vi "ElevatorSim_exampleX.vi"() -> ()   [LabVIEW 2019]
uses:
  <vilib>/Rock Robotics/WPI/ThirdParty/JAS_Junk/TrajLib/DCMOTOR.CTL
  <vilib>/Rock Robotics/WPI/ThirdParty/JAS_Junk/TrajLib/LINEAR_SYSTEM.ctl
  <vilib>/Analysis/Matrix/Datatypes/RealMatrix.ctl
  <vilib>/Rock Robotics/WPI/ThirdParty/JAS_Junk/TrajLib/LINEAR_QUADRATIC_REGULATOR.ctl
  <vilib>/Rock Robotics/WPI/ThirdParty/JAS_Junk/TrajLib/KALMAN_FILTER.ctl
  <vilib>/Rock Robotics/WPI/ThirdParty/JAS_Junk/TrajLib/LINEAR_SYSTEM_LOOP.ctl
  <vilib>/Rock Robotics/WPI/ThirdParty/JAS_Junk/TrajLib/LINEAR_PLANT_INV_FF.ctl
  <vilib>/Rock Robotics/WPI/ThirdParty/JAS_Junk/TrajLib/ELEVATOR_SIM.ctl
  <vilib>/Rock Robotics/WPI/ThirdParty/JAS_Junk/TrajLib/LINEAR_SYSTEM_SIM.ctl
  <vilib>/numeric/Random Number (Range) DBL.vi
  <vilib>/Rock Robotics/WPI/ThirdParty/JAS_Junk/TrajLib/MatBuilder_Create.vi
  <vilib>/Rock Robotics/WPI/ThirdParty/JAS_Junk/TrajLib/DCMotor_New.vi
  <vilib>/Rock Robotics/WPI/ThirdParty/JAS_Junk/TrajLib/Units_RotationsPerMinuteToRadiansPerSecond.vi
  <vilib>/Rock Robotics/WPI/ThirdParty/JAS_Junk/TrajLib/MatBuilder_Fill.vi
  <vilib>/Rock Robotics/WPI/ThirdParty/JAS_Junk/TrajLib/MatrixHelper_Zero.vi
  <vilib>/Rock Robotics/WPI/ThirdParty/JAS_Junk/TrajLib/LinearSystem_New.vi
  <vilib>/Rock Robotics/WPI/ThirdParty/JAS_Junk/TrajLib/Trajectory_Library.lvlib
  <vilib>/Analysis/Matrix/NI_Matrix.lvlib
panel:
  in  "Tab Control":T1(tab)
  out "Elevator Motor":T2 {"Jr_KgM2" format="%13.5p"; "L_H" format="%13.5p"; "Kt_NMPerAmp" format="%13.5p"; "KvINV_RadPerSecPerVolt" format="%13.5p"; "R_Ohms" format="%13.5p"; "FreeSpeed_RadPerSec" format="%13.5p"; "FreeCurrent_Amps" format="%13.5p"; "StallCurrent_Amps" format="%13.5p"; "StallTorque_NM" format="%13.5p"; "nominalVoltage_Volts" format="%13.5p"}
  out "m_Elevator":T3
  out "KalmanFilter":T5
  out "Kalman Error":bool
  out "LinearQuadraticRegulator":T6
  out "LQR Error":bool
  out "Linear System Loop":T7
  out "LinSysLoop_Error":bool
  out "Elevator Simulaation":T9 {"GearBox"."Jr_KgM2" format="%13.5p"; "GearBox"."L_H" format="%13.5p"; "GearBox"."Kt_NMPerAmp" format="%13.5p"; "GearBox"."KvINV_RadPerSecPerVolt" format="%13.5p"; "GearBox"."R_Ohms" format="%13.5p"; "GearBox"."FreeSpeed_RadPerSec" format="%13.5p"; "GearBox"."FreeCurrent_Amps" format="%13.5p"; "GearBox"."StallCurrent_Amps" format="%13.5p"; "GearBox"."StallTorque_NM" format="%13.5p"; "GearBox"."nominalVoltage_Volts" format="%13.5p"}
  out "Shooting A":T4
  out "Shooting B":T4
  out "Battery Voltage":dbl format="%20.3f"
  in  "Extra weight":bool
  out "CO Chart":cluster{dbl, "Voltage":dbl}(graph)
  in  "GO UP":bool
  out "Encoer Speed\nRad/Sec":dbl(slide) scale=-1.0..6.0
  out "Height":dbl format="%20.3f"
  out "Cor Err":bool
  out "Kalman Filtered\nHeight":dbl format="%20.3f"
  out "PV Chart":T11(graph)
  out "Predict Err":bool
  out "Motor Volt Dmd (CO)":dbl format="%20.3f"
  out "At Top":bool
  out "At Bottom":bool
  out "Motor Amps":dbl format="%20.3f"
  # "<States,States>"
  # "<States,Inputs>"
  # "<Outputs,States>"
  # "<Outputs,Inputs>"
  # "Steady State Gain  \n<States,Outputs>"
  # "State Estimate <Statess,1>"
  # "<States,States>"
  # "<States,Inputs>"
  # "<Outputs,States>"
  # "<Outputs,Inputs>"
  # "Ref State <States,1>"
  # "Comp and capped \noutput <Inputs,1>"
  # "Controller gain\n<Inputs,States>"
  # "<States,1>"
  # "<FUTURE --- CLAMP TYPE -- For now\nuse Normalize>"
  # "Steady State Gain  \n<States,Outputs>"
  # "State Estimate <Statess,1>"
  # "<States,States>"
  # "<States,Inputs>"
  # "<Outputs,States>"
  # "<Outputs,Inputs>"
  # "<States,1>"
  # "<Inputs,1>"
  # "<States,Inputs>"
  # "<States,States>"
  # "Ref State <States,1>"
  # "Comp and capped \noutput <Inputs,1>"
  # "Controller gain\n<Inputs,States>"
  # "<States, 1>"
  # "<Outputs, 1>"
  # "<Inputs, 1>"
  # "<Outputs, 1>"
  # "<States,States>"
  # "<States,Inputs>"
  # "<Outputs,States>"
  # "<Outputs,Inputs>"
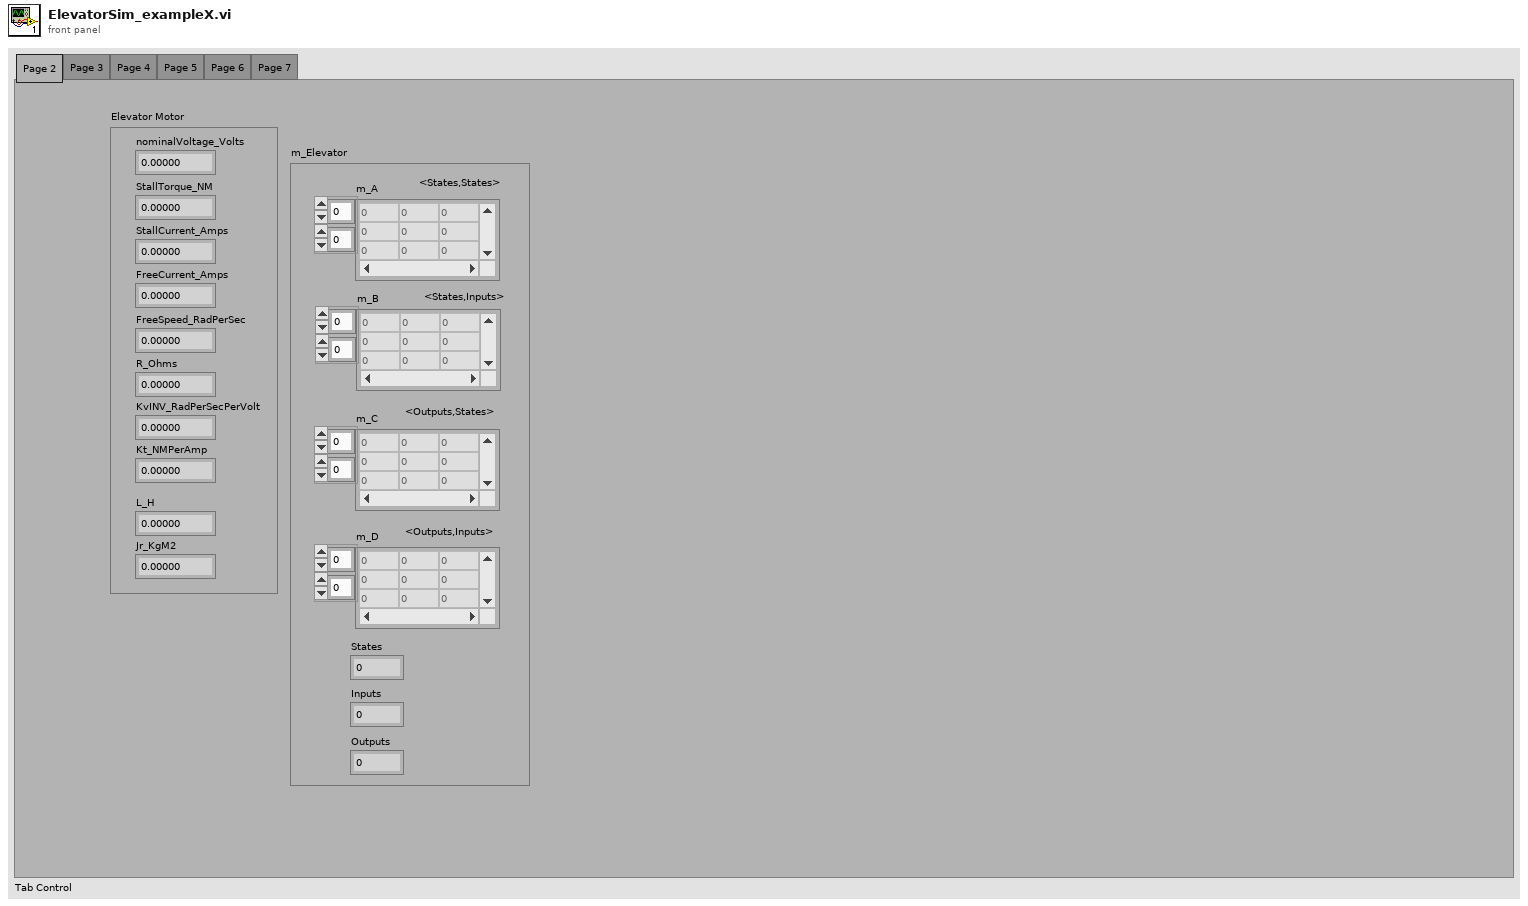
[diagram p1: front panel]
types:
  T1 = enum32{"Page 2", "Page 3", "Page 4", "Page 5", "Page 6", "Page 7"}
  T2 = typedef "Trajectory_Library.lvlib/DCMOTOR.CTL" = cluster{"nominalVoltage_Volts":dbl, "StallTorque_NM":dbl, "StallCurrent_Amps":dbl, "FreeCurrent_Amps":dbl, "FreeSpeed_RadPerSec":dbl, "R_Ohms":dbl, "KvINV_RadPerSecPerVolt":dbl, "Kt_NMPerAmp":dbl, "L_H":dbl, "Jr_KgM2":dbl}
  T3 = typedef "Trajectory_Library.lvlib/LINEAR_SYSTEM.ctl" = cluster{"m_A":T4, "m_B":T4, "m_C":T4, "m_D":T4, "States":i32, "Inputs":i32, "Outputs":i32}
  T4 = typedef "NI_Matrix.lvlib/RealMatrix.ctl" = dbl[][]
  T5 = typedef "Trajectory_Library.lvlib/KALMAN_FILTER.ctl" = cluster{"m_K":T4, "m_xHat":T4, "States":i32, "Outputs":i32, "m_Plant":T3}
  T6 = typedef "Trajectory_Library.lvlib/LINEAR_QUADRATIC_REGULATOR.ctl" = cluster{"m_r":T4, "m_U":T4, "m_K":T4, "States":i32, "Inputs":i32}
  T7 = typedef "Trajectory_Library.lvlib/LINEAR_SYSTEM_LOOP.ctl" = cluster{"Controller":T6, "FeedForward":T8, "Observer":T5, "Next_R":T4, "Clamp Max":T4}
  T8 = typedef "Trajectory_Library.lvlib/LINEAR_PLANT_INV_FF.ctl" = cluster{"m_R":T4, "m_Uff":T4, "m_B":T4, "m_A":T4, "States":i32, "Inputs":i32}
  T9 = typedef "Trajectory_Library.lvlib/ELEVATOR_SIM.ctl" = cluster{"LinearSystemSim":T10, "GearBox":T2, "Gearing":dbl, "DrumRadius_M":dbl, "MinHeight_M":dbl, "MaxHeight_M":dbl, "CarriageMass_Kg":dbl}
  T10 = typedef "Trajectory_Library.lvlib/LINEAR_SYSTEM_SIM.ctl" = cluster{"m_Plant":T3, "m_X":T4, "m_Y":T4, "m_U":T4, "MeasureStdDev":T4}
  T11 = cluster{"upper limit":dbl, "Real Matrix Element":dbl, "Real Matrix Element":dbl}
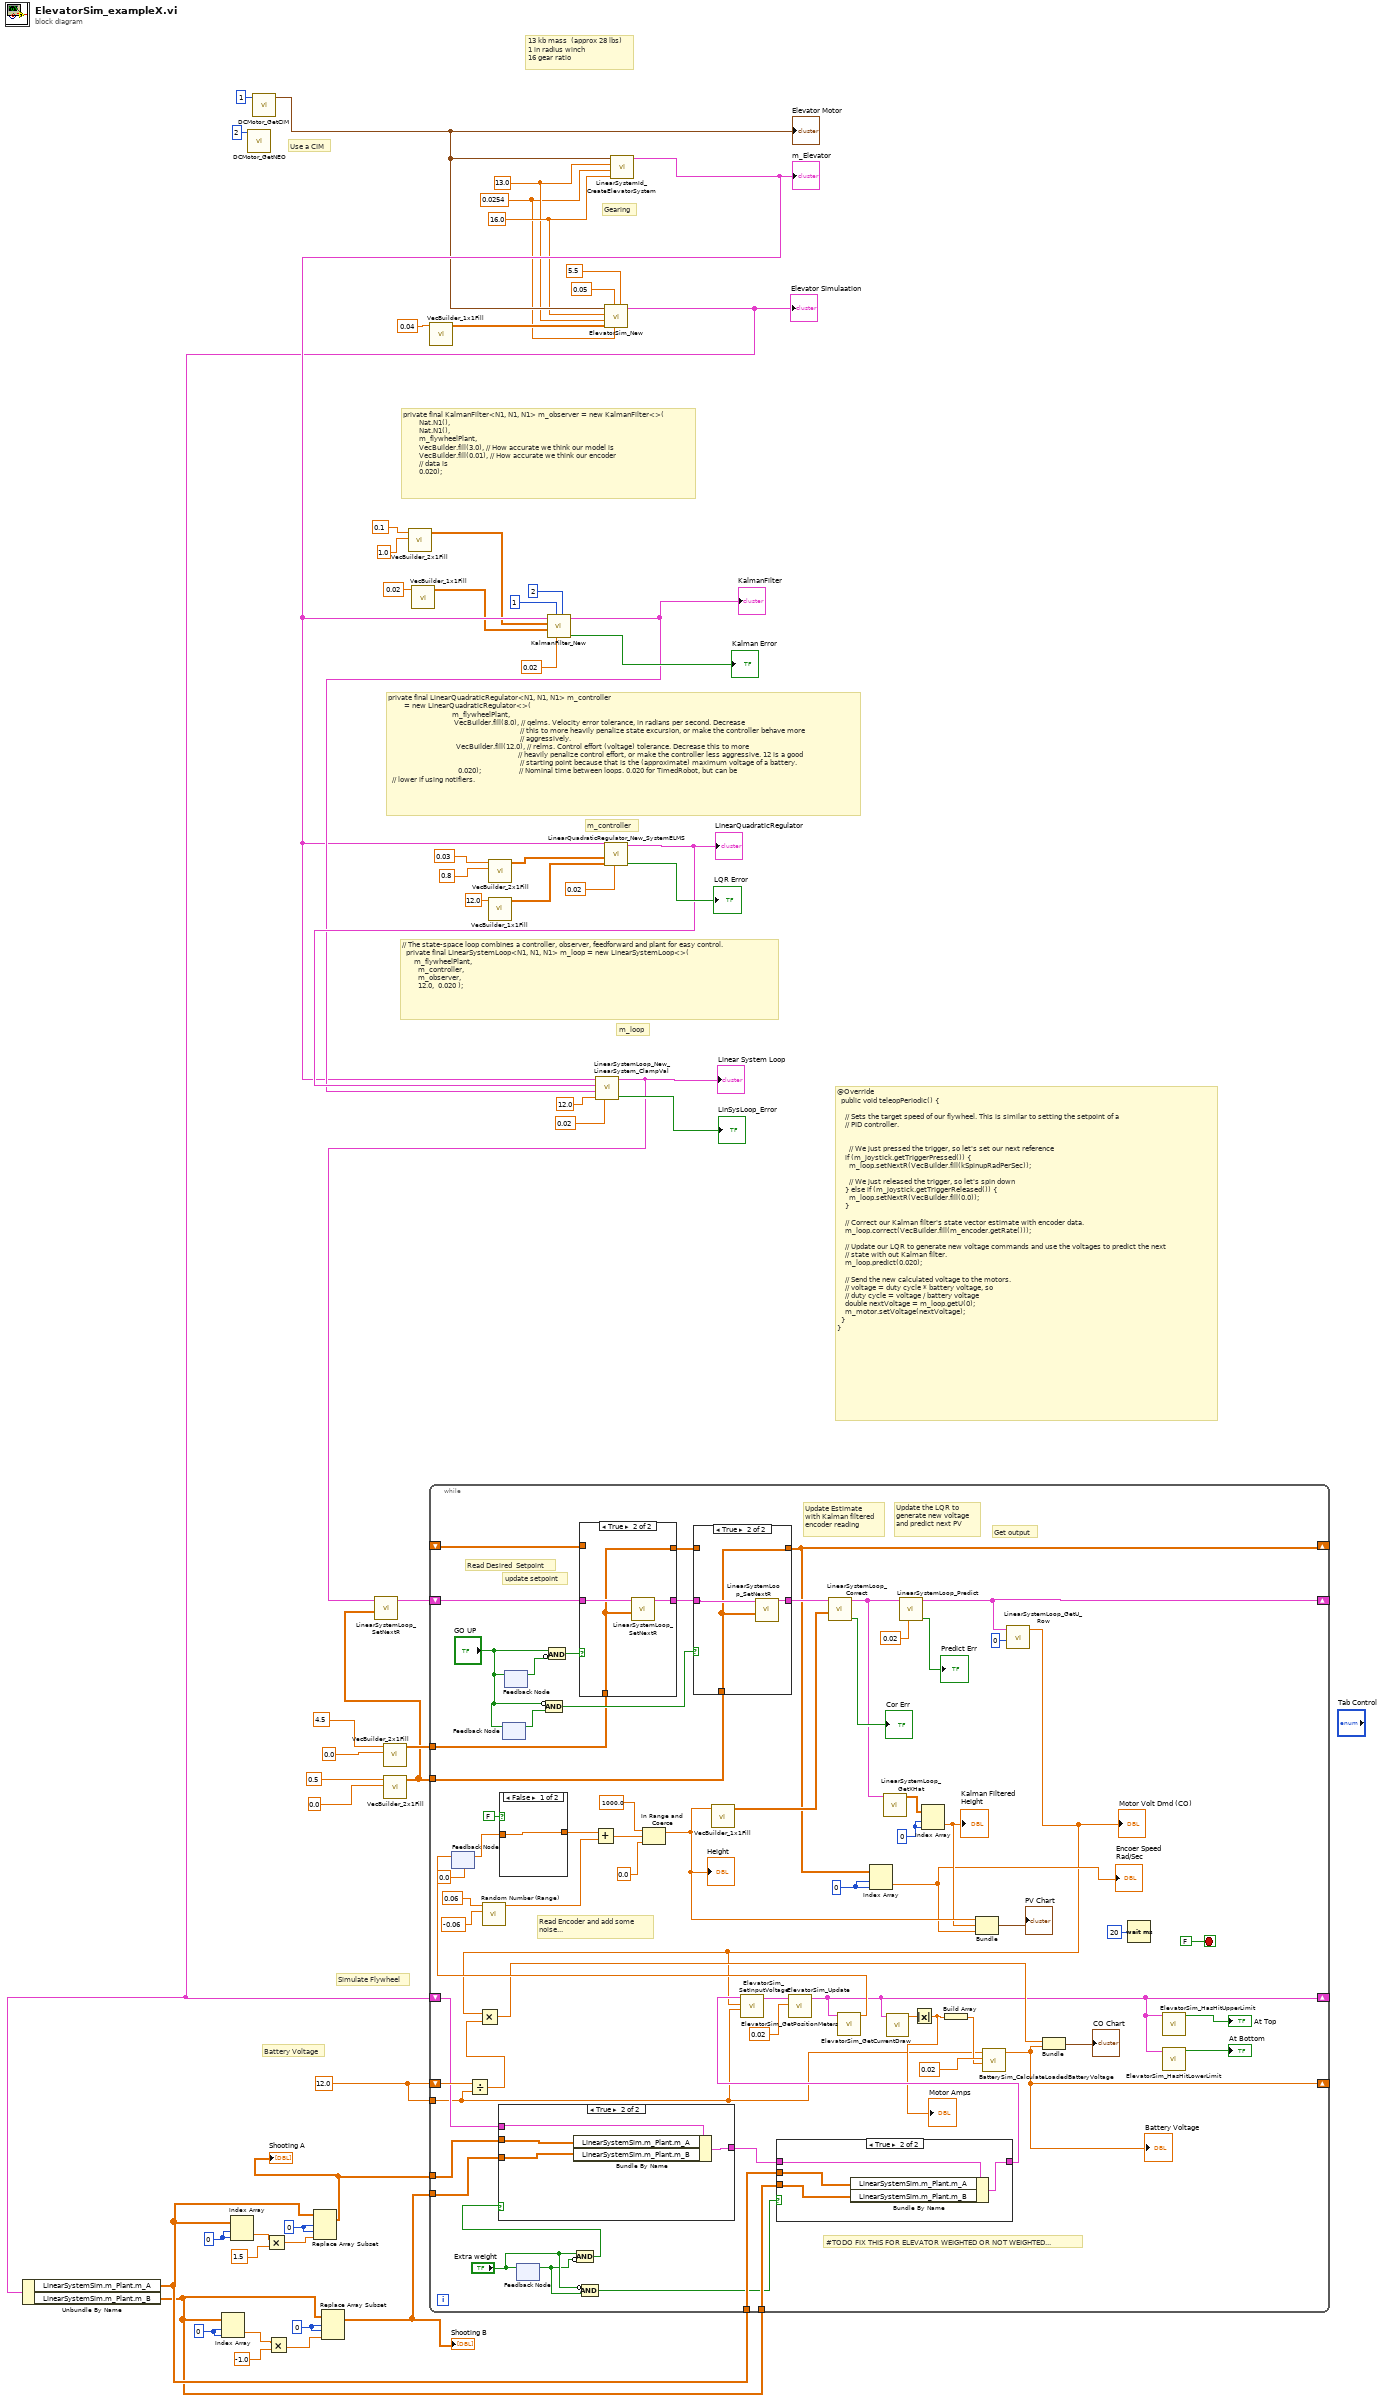
[diagram p0: block diagram]
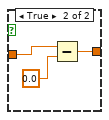
[diagram p4: hidden frame]
diagram:
  w13 = 0 ("index (row)")
  w14 = 0 ("index (row)")
  w15 = 0 ("index (row)")
  w16 = 0 ("index (row)")
  w36 = 16.0 ("G")
  w34 = 0.0254 ("radiusMeters")
  w35 = 13.0 ("massKg")
  w48 = 12.0
  # "Simulate Flywheel"
  # "m_loop"
  # "m_controller"
  # "13 kb mass  (approx 28 lbs)\n1 in radius winch\n16 gear ratio"
  # "Gearing"
  # "Use a CIM"
  # "Battery Voltage"
  # "@Override\n  public void teleopPeriodic() {\n\n    // Sets the target speed of our flywheel. This is similar to setting the setpoint of a\n    // PID controller.\n\n\n      // We just pressed the trigger, so let's set our next reference\n    if (m_joystick.getTriggerPressed()) {\n      m_loop.setNextR(VecBuilder.fill(kSpinupRadPerSec));\n\n      // We just released the trigger, so let's spin down\n    } else if (m_joystick.getTriggerReleased()) {\n      m_loop.setNextR(VecBuilder.fill(0.0));\n    }\n\n    // Correct our Kalman filter's state vector estimate with encoder data.\n    m_loop.correct(VecBuilder.fill(m_encoder.getRate()));\n\n    // Update our LQR to generate new voltage commands and use the voltages to predict the next\n    // state with out Kalman filter.\n    m_loop.predict(0.020);\n\n    // Send the new calculated voltage to the motors.\n    // voltage = duty cycle * battery voltage, so\n    // duty cycle = voltage / battery voltage\n    double nextVoltage = m_loop.getU(0);\n    m_motor.setVoltage(nextVoltage);\n  }\n}"
  # "// The state-space loop combines a controller, observer, feedforward and plant for easy control.\n  private final LinearSystemLoop<N1, N1, N1> m_loop = new LinearSystemLoop<>(\n      m_flywheelPlant,\n        m_controller,\n        m_observer,\n        12.0,  0.020 );"
  # "private final LinearQuadraticRegulator<N1, N1, N1> m_controller\n        = new LinearQuadraticRegulator<>(\n                                m_flywheelPlant,\n                                 VecBuilder.fill(8.0), // qelms. Velocity error tolerance, in radians per second. Decrease\n                                                                  // this to more heavily penalize state excursion, or make the controller behave more\n                                                                  // aggressively.\n                                  VecBuilder.fill(12.0), // relms. Control effort (voltage) tolerance. Decrease this to more\n                                                                 // heavily penalize control effort, or make the controller less aggressive. 12 is a good\n                                                                  // starting point because that is the (approximate) maximum voltage of a battery.\n                                   0.020);                   // Nominal time between loops. 0.020 for TimedRobot, but can be\n  // lower if using notifiers."
  # "private final KalmanFilter<N1, N1, N1> m_observer = new KalmanFilter<>(\n        Nat.N1(), \n        Nat.N1(),\n        m_flywheelPlant,\n        VecBuilder.fill(3.0), // How accurate we think our model is\n        VecBuilder.fill(0.01), // How accurate we think our encoder\n        // data is\n        0.020);"
  n1 = call <vilib>:"DCMotor_GetNEO.vi"("Num Motors"=2) -> ()  [unwired: 10 in, 1 out]
  n2 = call <vilib>:"DCMotor_GetCIM.vi"("Num Motors"=1) -> ("DCMOTOR"=w41:T2)  [unwired: 10 in]
  "Elevator Motor" <- w41
  n3 = call <vilib>:"VecBuilder_2x1Fill.vi"("R1"=0.0, "R0"=4.5 ("RotationsPerMinute")) -> ("output matrix"=w6:T4)  [unwired: 9 in]
  n4 = call <vilib>:"VecBuilder_2x1Fill.vi"("R1"=0.0, "R0"=0.5 ("R0_C0")) -> ("output matrix"=w1:T4)  [unwired: 9 in]
  n5 = call <vilib>:"VecBuilder_2x1Fill.vi"("R1"=1.0, "R0"=0.1 ("R0_C0")) -> ("output matrix"=w27:T4)  [unwired: 9 in]
  n6 = call <vilib>:"VecBuilder_1x1Fill.vi"("R0_C0"=0.02) -> ("output matrix"=w26:T4)  [unwired: 10 in]
  n7 = call <vilib>:"VecBuilder_1x1Fill.vi"("R0_C0"=0.04) -> ("output matrix"=w37:T4)  [unwired: 10 in]
  n8 = call <vilib>:"VecBuilder_1x1Fill.vi"("R0_C0"=12.0) -> ("output matrix"=w20:T4)  [unwired: 10 in]
  n9 = call <vilib>:"VecBuilder_2x1Fill.vi"("R1"=0.8 ("R0_C0"), "R0"=0.03 ("R0_C0")) -> ("output matrix"=w22:T4)  [unwired: 9 in]
  n10 = call <vilib>:"ElevatorSim_New.vi"("MaxHeight_Meters"=5.5, "DrumRadius_Meters"=w34, "MinHeight_Meters"=0.05, "MeasurementStdDev"=w37, "CarriageMass_Kg"=w35, "Gearing"=w36, "GearBox"=w41) -> ("ElevatorSim"=w40:T9)  [unwired: 3 in, 1 out]
  "Elevator Simulaation" <- w40
  n11 = Unbundle By Name(w40) -> ("LinearSystemSim.m_Plant.m_A"=w46:T4, "LinearSystemSim.m_Plant.m_B"=w45:T4)
  n12 = Index Array(array=w45, index (row)=w16, index (col)=w16) -> (element=w8:dbl)
  n13 = Index Array(array=w46, index (row)=w15, index (col)=w15) -> (element=w12:dbl)
  n14 = Multiply(x=w12, y=1.5) -> (x*y=w10:dbl)
  n15 = Multiply(x=w8, y=-1.0) -> (x*y=w7:dbl)
  n16 = Replace Array Subset(array=w46, new element=w10, index (row)=w13, index (col)=w13) -> (w44:T4)
  "Shooting A" <- w44
  n17 = Replace Array Subset(array=w45, new element=w7, index (row)=w14, index (col)=w14) -> (w43:T4)
  "Shooting B" <- w43
  n18 = call <vilib>:"LinearSystemId_CreateElevatorSystem.vi"("G"=w36, "radiusMeters"=w34, "massKg"=w35, "DCMOTOR"=w41) -> ("Linearsystem"=w42:T3)  [unwired: 6 in, 1 out]
  "m_Elevator" <- w42
  n19 = call <vilib>:"KalmanFilter_New.vi"("States"=2, "dt_Seconds"=0.02, "Outputs"=1, "MeasurementStdDevs"=w26, "StateStdDevs"=w27, "Plant"=w42) -> ("Error"=→"Kalman Error":bool, "KalmanFilter"=w52:T5)  [unwired: 4 in]
  "KalmanFilter" <- w52
  n20 = call <vilib>:"LinearQuadraticRegulator_New_SystemELMS.vi"("dt_Seconds"=0.02, "Relms"=w20, "Qelms"=w22, "LINEARSYSTEM"=w42) -> ("Error"=→"LQR Error":bool, "LinearQuadraticRegulator"=w53:T6)  [unwired: 6 in]
  "LinearQuadraticRegulator" <- w53
  n21 = call <vilib>:"LinearSystemLoop_New_LinearSystem_ClampVal.vi"("dT_Seconds"=0.02, "Max_Voltage"=12.0, "Observer"=w52, "Controller"=w53, "Plant"=w42) -> ("Error"=→"LinSysLoop_Error":bool, "Linear System Loop"=w2:T7)  [unwired: 5 in]
  "Linear System Loop" <- w2
  n22 = call <vilib>:"LinearSystemLoop_SetNextR.vi"("R"=w1, "input inear System Loop"=w2) -> ("out Linear System Loop"=w3:T7)  [unwired: 8 in, 1 out]
  n23 = while {
    shift-right: [w67] -> _
    shift-left: w3 -> [w116]
    tunnel: w6 -> [w114]
    tunnel: w1 -> [w113]
    shift-right: [w66] -> _
    shift-left: w40 -> [w76]
    shift-right: [w88] -> _
    shift-left: _ -> [w89]
    shift-right: [w78] -> _
    shift-left: w48 -> [w83]
    tunnel: w48 -> [w57]
    tunnel: w46 -> [w71]
    tunnel: w45 -> [w70]
    tunnel: w44 -> [w69]
    tunnel: w43 -> [w68]
    stop <- FALSE stop-if-true
    w87 = 0 ("index (row)")
    w103 = 0 ("index (row)")
    # "#TODO FIX THIS FOR ELEVATOR WEIGHTED OR NOT WEIGHTED..."
    # "Get output"
    # "Update the LQR to \ngenerate new voltage\nand predict next PV"
    # "update setpoint"
    # "Read Desired  Setpoint"
    # "Update Estimate\nwith Kalman filtered\nencoder reading"
    # "Read Encoder and add some \nnoise..."
    n24 = feedback #1(0.0 ("Velocity_RadPerSec")) -> (w85:dbl)
    n25 = Divide(x=w83, y=w57) -> (x/y=w82:dbl)
    n26 = call-poly <vilib>:"Random Number (Range).vi"("lower bound (0)"=-0.06, "upper bound (100)"=0.06) -> ("number"=w110:dbl)  [unwired: 9 in]
    n27 = case shown="False" FALSE {
      tunnel: w85 -> [w134 w137]
      tunnel: [w134 w136] -> w84
      frame False {
      }
      frame True {
        n28 = Subtract(x=w137, y=0.0) -> (x-y=w136:dbl)
      }
    }
    n29 = feedback #2() -> (w120:bool)  [unwired: 1 in]
    n30 = feedback-in #2("GO UP") -> ()
    n31 = feedback-in #3("GO UP") -> ()
    n32 = feedback #3() -> (w121:bool)  [unwired: 1 in]
    n33 = feedback-in #4("Extra weight") -> ()
    n34 = feedback #4() -> (w62:bool)  [unwired: 1 in]
    n35 = Compound Arithmetic op=AND(invert "GO UP", w120) -> (w117:bool)
    n36 = Compound Arithmetic op=AND("GO UP", invert w121) -> (w118:bool)
    n37 = Compound Arithmetic op=AND("Extra weight", invert w62) -> (w72:bool)
    n38 = case shown="True" w72 {
      tunnel: w76 -> [w129 w133]
      tunnel: [w129 w130] -> w75
      tunnel: w69 -> [_ w132]
      tunnel: w68 -> [_ w131]
      frame False {
      }
      frame True {
        n39 = Bundle By Name(cluster=w133, "LinearSystemSim.m_Plant.m_A"=w132, "LinearSystemSim.m_Plant.m_B"=w131) -> (w130:T9)
      }
    }
    n40 = case shown="True" w118 {
      tunnel: w116 -> [w144 w146]
      tunnel: [w144 w147] -> w115
      tunnel: w114 -> [_ w145]
      tunnel: [w143 w145] -> w90
      tunnel: w89 -> [w143 _]
      frame False {
      }
      frame True {
        n41 = call <vilib>:"LinearSystemLoop_SetNextR.vi"("R"=w145, "input inear System Loop"=w146) -> ("out Linear System Loop"=w147:T7)  [unwired: 8 in, 1 out]
      }
    }
    n42 = Compound Arithmetic op=AND(invert "Extra weight", w62) -> (w61:bool)
    n43 = Add(x=w84, y=w110) -> (x+y=w108:dbl)
    n44 = In Range and Coerce(upper limit=1000.0, x=w108, lower limit=0.0) -> (coerced(x)=w101:dbl)  [unwired: 1 out]
    "Height" <- w101
    n45 = case shown="True" w117 {
      tunnel: w115 -> [w139 w141]
      tunnel: [w139 w142] -> w106
      tunnel: w113 -> [_ w140]
      tunnel: w90 -> [w138 _]
      tunnel: [w138 w140] -> w88
      frame False {
      }
      frame True {
        n46 = call <vilib>:"LinearSystemLoop_SetNextR.vi"("R"=w140, "input inear System Loop"=w141) -> ("out Linear System Loop"=w142:T7)  [unwired: 8 in, 1 out]
      }
    }
    n47 = call <vilib>:"VecBuilder_1x1Fill.vi"("R0_C0"=w101) -> ("output matrix"=w105:T4)  [unwired: 10 in]
    n48 = case shown="True" w61 {
      tunnel: w75 -> [w124 w128]
      tunnel: [w124 w127] -> w74
      tunnel: w71 -> [_ w126]
      tunnel: w70 -> [_ w125]
      frame False {
      }
      frame True {
        n49 = Bundle By Name(cluster=w128, "LinearSystemSim.m_Plant.m_A"=w126, "LinearSystemSim.m_Plant.m_B"=w125) -> (w127:T9)
      }
    }
    n50 = call <vilib>:"LinearSystemLoop_Correct.vi"("Y"=w105, "input inear System Loop"=w106) -> ("Error"=→"Cor Err":bool, "out Linear System Loop"=w98:T7)  [unwired: 8 in]
    n51 = Index Array(array=w88, index (row)=w87, index (col)=w87) -> (element=w86:dbl)
    "Encoer Speed\nRad/Sec" <- w86
    n52 = call <vilib>:"LinearSystemLoop_GetXHat.vi"("input inear System Loop"=w98) -> ("XHat"=w102:T4)  [unwired: 10 in]
    n53 = call <vilib>:"LinearSystemLoop_Predict.vi"("dT_Seconds"=0.02, "input inear System Loop"=w98) -> ("Error"=→"Predict Err":bool, "out Linear System Loop"=w67:T7)  [unwired: 8 in]
    n54 = Index Array(array=w102, index (row)=w103, index (col)=w103) -> (element=w100:dbl)
    "Kalman Filtered\nHeight" <- w100
    n55 = Bundle("upper limit"=w101, "Real Matrix Element"=w100, "Real Matrix Element"=w86) -> (→"PV Chart":T11)  [unwired: 1 in]
    n56 = call <vilib>:"LinearSystemLoop_GetU_Row.vi"("Row"=0, "input inear System Loop"=w67) -> ("U"=w58:dbl)  [unwired: 9 in]
    "Motor Volt Dmd (CO)" <- w58
    n57 = Multiply(x=w58, y=w82) -> (x*y=w77:dbl)
    n58 = call <vilib>:"ElevatorSim_SetInputVoltage.vi"("Battery_Volts"=w57, "Input_Voltage"=w58, "in ElevatorSim"=w74) -> ("out ElevatorSim"=w94:T9)  [unwired: 8 in]
    n59 = call <vilib>:"ElevatorSim_Update.vi"("dT_Seconds"=0.02, "in ElevatorSim"=w94) -> ("out ElevatorSim"=w66:T9)  [unwired: 8 in, 1 out]
    n60 = call <vilib>:"ElevatorSim_GetPositionMeters.vi"("ElevatorSim"=w66) -> ("Position_Meters"=w92:dbl)  [unwired: 10 in]
    n61 = feedback-in #1(w92) -> ()
    n62 = call <vilib>:"ElevatorSim_GetCurrentDraw.vi"("ElevatorSim"=w66) -> ("Current_Amps"=w60:dbl)  [unwired: 10 in]
    n63 = Absolute Value(x=w60) -> (abs(x)=w59:dbl)
    "Motor Amps" <- w59
    n64 = Build Array(w59) -> (w80:dbl[])
    n65 = call <vilib>:"BatterySim_CalculateLoadedBatteryVoltage.vi"("Currents"=w80, "Resistance_Ohms"=0.02, "NominalVoltage"=w57) -> ("Voltage"=w78:dbl)  [unwired: 8 in]
    "Battery Voltage" <- w78
    n66 = Bundle(w77, "Voltage"=w78) -> (→"CO Chart":cluster{dbl, "Voltage":dbl})  [unwired: 1 in]
    n67 = Wait (ms)(milliseconds to wait=u32 20) -> ()  [unwired: 1 out]
    n68 = call <vilib>:"ElevatorSim_HasHitUpperLimit.vi"("ElevatorSim"=w66) -> ("At HIgh LImit"=→"At Top":bool)  [unwired: 10 in]
    n69 = call <vilib>:"ElevatorSim_HasHitLowerLimit.vi"("ElevatorSim"=w66) -> ("AtLowLimit"=→"At Bottom":bool)  [unwired: 10 in]
  }
